vi "Write FIFO.vi"   [LabVIEW 2011, in "FIFO.lvlib"]
uses:
  <instrlib>/RF-RIO/FIFO/FIFO/FPGA/FIFO.lvlib
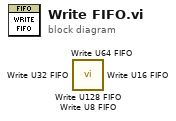
[diagram p0: block diagram]
diagram:
  n1 = call <instrlib>:"Write U128 FIFO.vi"() -> ()  [unwired: 15 in, 1 out]
  n2 = call <instrlib>:"Write U64 FIFO.vi"() -> ()  [unwired: 15 in, 1 out]
  n3 = call <instrlib>:"Write U32 FIFO.vi"() -> ()  [unwired: 15 in, 1 out]
  n4 = call <instrlib>:"Write U16 FIFO.vi"() -> ()  [unwired: 15 in, 1 out]
  n5 = call <instrlib>:"Write U8 FIFO.vi"() -> ()  [unwired: 15 in, 1 out]
